vi "Update UI Project.vi"(8 "error in (no error)":errorcluster, 10 "New Name":string, 11 "Template Project Path":path) -> (0 "error out":errorcluster)   [LabVIEW 2021, in "Plugin Generator.lvlib"]
uses:
  Plugin Generator.lvlib
  <vilib>/CIF Foundation/CIF LabVIEW Scripting/LV Scripting/LV Scripting Utilities.lvlib
  <vilib>/CIF Foundation/CIF Utilities/File/File_CIF_U.lvlib
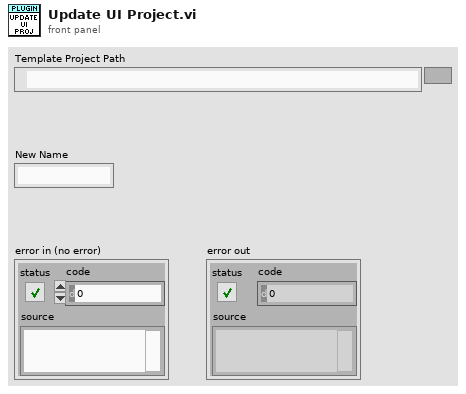
[diagram p1: front panel]
types:
  T1 = cluster{"Library Name":string, "Update Folder Name":bool}[]
  T2 = typedef "LV Scripting Utilities.lvlib/Target References.ctl" = cluster{"Target Reference":refnum<vi>, "VI References":refnum<vi>[], "Library References":refnum<vi>[], "Build References":refnum<vi>[]}
  T3 = typedef "LV Scripting Utilities.lvlib/Library Map.ctl" = map{string, refnum<vi>}
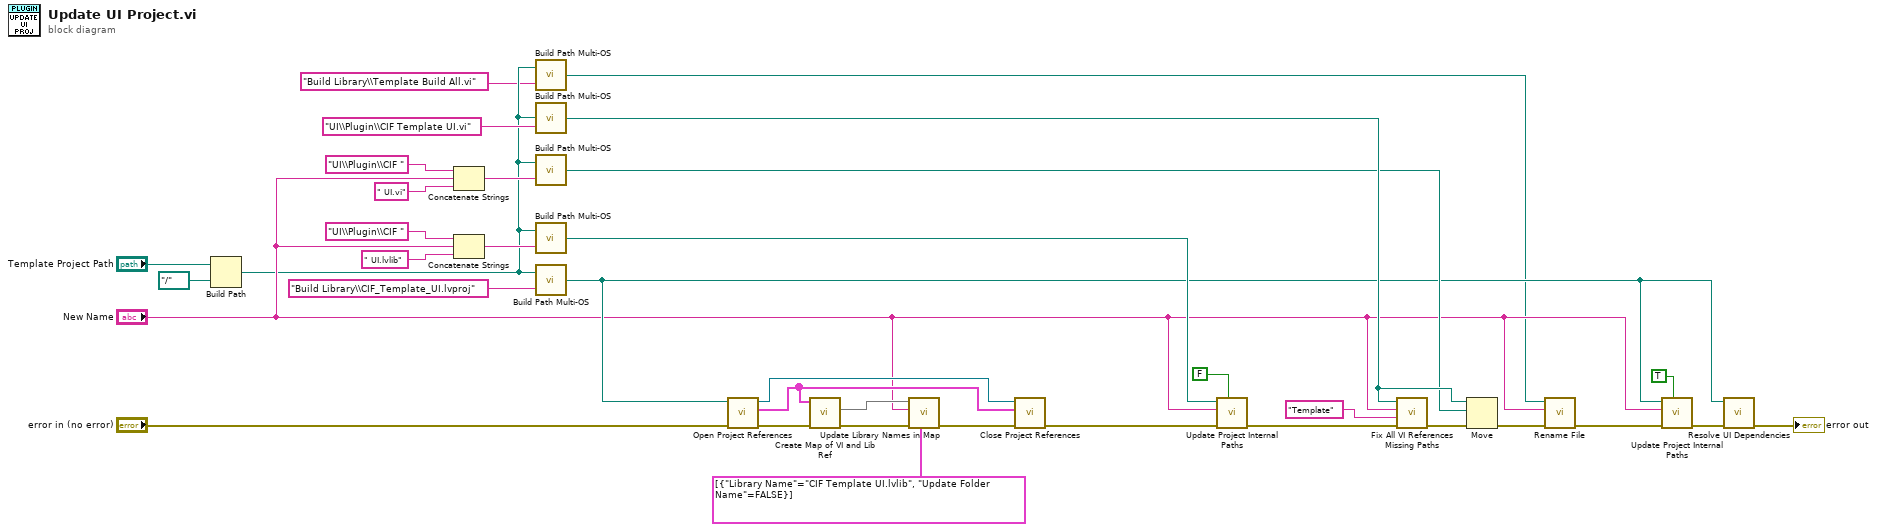
[diagram p0: block diagram]
diagram:
  n1 = Build Path(base path="Template Project Path", name or relative path=path "../..") -> (appended path=w3:path)
  n2 = Concatenate Strings("UI\\Plugin\\CIF " ("Class Name"), "New Name", " UI.vi" ("Class Name")) -> (w29:string)
  n3 = Concatenate Strings("UI\\Plugin\\CIF " ("Class Name"), "New Name", " UI.lvlib" ("Class Name")) -> (w18:string)
  n4 = call <vilib>:"Build Path Multi-OS.vi"("name or relative path"="Build Library\\Template Build All.vi" ("Class Name"), "base path"=w3) -> ("appended path"=w1:path)
  n5 = call <vilib>:"Build Path Multi-OS.vi"("name or relative path"="UI\\Plugin\\CIF Template UI.vi" ("Class Name"), "base path"=w3) -> ("appended path"=w32:path)
  n6 = call <vilib>:"Build Path Multi-OS.vi"("name or relative path"=w29, "base path"=w3) -> ("appended path"=w28:path)
  n7 = call <vilib>:"Build Path Multi-OS.vi"("name or relative path"=w18, "base path"=w3) -> ("appended path"=w25:path)
  n8 = call <vilib>:"Build Path Multi-OS.vi"("name or relative path"="Build Library\\CIF_Template_UI.lvproj" ("Class Name"), "base path"=w3) -> ("appended path"=w7:path)
  n9 = call <vilib>:"Open Project References.vi"("error in"="error in (no error)", "Project Path"=w7) -> ("error out"=w12:errorcluster, "VI, Library, and Build References"=w9:T2[], "Project Reference"=w8:refnum<vi>)  [unwired: 7 in]
  n10 = call <vilib>:"Create Map of VI and Lib Ref.vi"("error in"=w12, "VI, Library, and Build References"=w9) -> ("error out"=w22:errorcluster, "Library Map"=w23:T3)  [unwired: 6 in, 2 out]
  n11 = call <vilib>:"Update Library Names in Map.vi"("Libraries"=T1 [{"Library Name"="CIF Template UI.lvlib", "Update Folder Name"=FALSE}], "error in"=w22, "New Subname"="New Name", "Library Map"=w23) -> ("error out"=w11:errorcluster)  [unwired: 6 in, 1 out]
  n12 = call <vilib>:"Close Project References.vi"("error in"=w11, "VI, Library, and Build References"=w9, "Project Reference"=w8) -> ("error out"=w10:errorcluster)  [unwired: 8 in]
  n13 = call <vilib>:"Update Project Internal Paths.vi"("Rename Project"=FALSE, "error in (no error)"=w10, "New Subname"="New Name", "Project Path"=w25) -> ("error out"=w27:errorcluster)  [unwired: 7 in]
  n14 = call <vilib>:"Fix All VI References Missing Paths.vi"("error in (no error)"=w27, "Replace Subname"="Template" ("Subname to Replace"), "New Subname"="New Name", "VI Path"=w32) -> ("error out"=w26:errorcluster)  [unwired: 7 in]
  n15 = Move(source path=w32, error in=w26, 10:w28) -> (error out=w6:errorcluster)  [unwired: 2 in, 2 out]
  n16 = call "Rename File.vi"("error in (no error)"=w6, "New Subname"="New Name", "VI Path"=w1) -> ("error out"=w5:errorcluster)  [unwired: 8 in]
  n17 = call <vilib>:"Update Project Internal Paths.vi"("Rename Project"=TRUE, "error in (no error)"=w5, "New Subname"="New Name", "Project Path"=w7) -> ("error out"=w15:errorcluster)  [unwired: 7 in]
  n18 = call "Resolve UI Dependencies.vi"("error in"=w15, "Template Project Path"=w7) -> ("error out"=→"error out":errorcluster)  [unwired: 9 in]
